vi "DataSelector.vi"(0 "Number in":string, 5 "String in":string) -> (4 "String out":string, 6 "Number out":string)   [LabVIEW 2015]
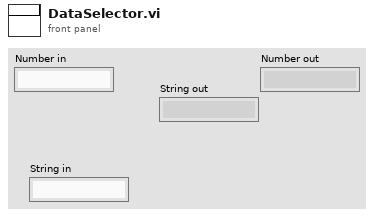
[diagram p1: front panel]
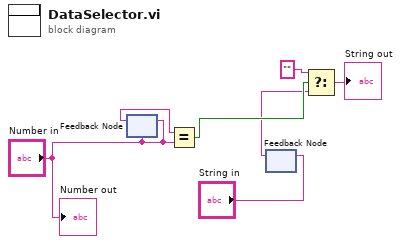
[diagram p0: block diagram]
diagram:
  n1 = feedback #1("Number in") -> (w2:string)
  n2 = feedback-in #1("Number in") -> ()
  n3 = Equal?(x=w2, y="Number in") -> (x = y?=w5:bool)
  n4 = feedback #2() -> (w3:string)  [unwired: 1 in]
  n5 = feedback-in #2("String in") -> ()
  n6 = Select(t="", s=w5, f=w3) -> (s? t:f=→"String out":string)
  "Number out" <- "Number in"
